vi "Populate Subpanels.vi"(8 "error in (no error)":errorcluster, 9 "View Labels (optional)":string[](array[string]), 10 "Views":refnum<class "Message Enqueuer.lvclass">[](array[class]), 11 "LeftListboxViewManager In":refnum<class "LeftListboxViewManager.lvclass">) -> (0 "error out":errorcluster, 3 "LeftListboxViewManager Out":refnum<class "LeftListboxViewManager.lvclass">)   [LabVIEW 2015, in "LeftListboxViewManager.lvlib" / "LeftListboxViewManager.lvclass"]
doc: "<License>\nCopyright © 2017 Composed Systems, LLC | All rights reserved\nwww.composed.io\n\nAuthor: Ethan Stern <ethan.stern@composed.io>\n\nThis software is provided \"AS IS\" WITHOUT WARRANTIES, either express or implied, AND IS FOR EDUCATIONAL PURPOSES ONLY.\n</License>"
uses:
  LeftListboxViewManager.lvclass
  <vilib>/ActorFramework/Message Enqueuer/Message Enqueuer.lvclass
  LeftListboxViewManager.lvclass/LeftListboxViewManager.ctl
  Framework/IViewable/IViewable Messages/Insert View Msg/Insert View Msg.lvclass/Insert View Msg.ctl
  <vilib>/ActorFramework/Message Enqueuer/Message Enqueuer.lvclass/Message Enqueuer.ctl
  <vilib>/ActorFramework/Message Enqueuer/Enqueue.vi
  <vilib>/ActorFramework/Message Priority Queue/Priority Enqueue.vi
  Framework/IViewManager/IViewManager/IViewManager.lvclass
  Framework/IViewable/IViewable Messages/Insert View Msg/Insert View Msg.lvclass
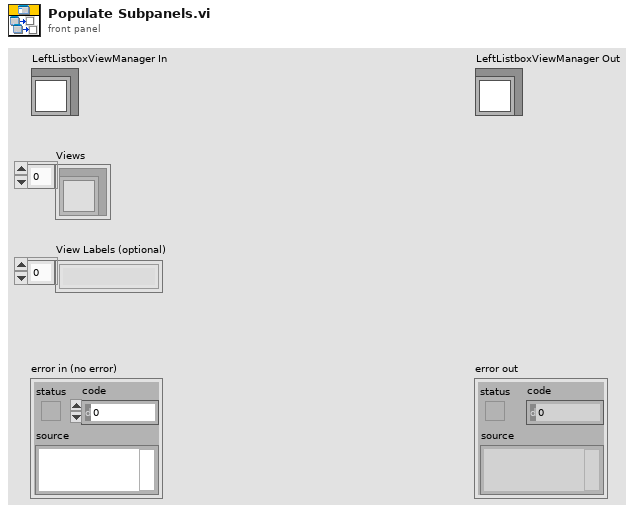
[diagram p1: front panel]
types:
  T1 = typedef "ProtectedSubpanel.lvlib/ProtectedSubpanel.lvclass/Protected Subpanel Reference.ctl" = refnum<data-value>
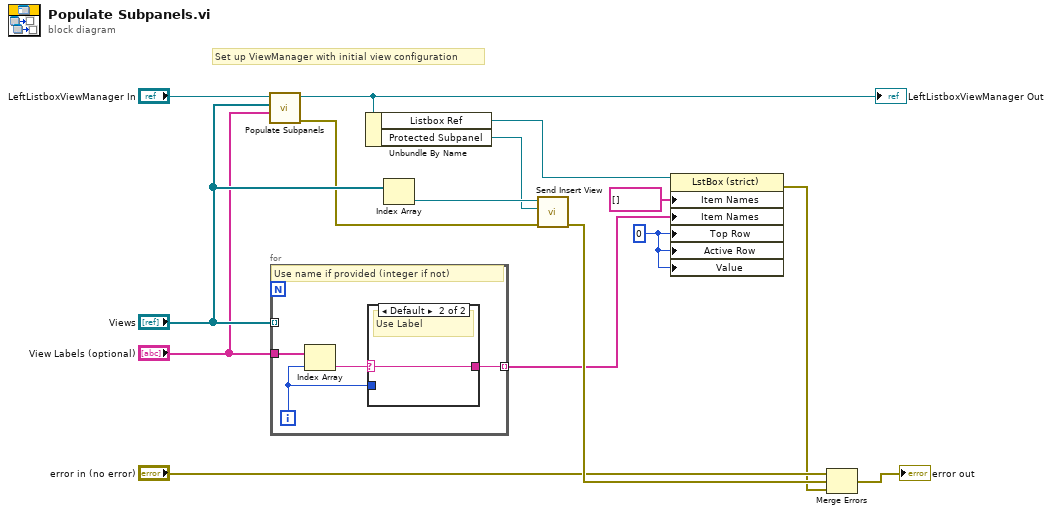
[diagram p0: block diagram]
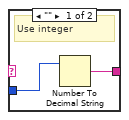
[diagram p2: hidden frame]
diagram:
  w5 = 0 ("Top Row")
  # "Set up ViewManager with initial view configuration"
  n1 = call-parent "Populate Subpanels.vi"("View Labels (optional)"="View Labels (optional)", "Views"="Views", "IViewManager In"="LeftListboxViewManager In") -> ("error out"=w2:errorcluster, "IViewManager Out"=w8:refnum<class "LeftListboxViewManager.lvclass">)  [unwired: 7 in]
  "LeftListboxViewManager Out" <- w8
  n2 = for {
    tunnel: "Views" -> [_] mode=indexing
    tunnel: "View Labels (optional)" -> [w19]
    tunnel: [w17] -> w3 mode=indexing
    i -> [w16]
    # "Use name if provided (integer if not)"
    n3 = Index Array(array=w19, index=w16) -> (element=w18:string)
    n4 = case shown="Default" w18 {
      selector: w18 -> [_ w22]
      tunnel: [w20 w22] -> w17
      tunnel: w16 -> [w21 _]
      frame "" {
        # "Use integer"
        n5 = Number To Decimal String(number=w21) -> (decimal integer string=w20:string)  [unwired: 1 in]
      }
      frame Default {
        # "Use Label"
      }
    }
  }
  n6 = Unbundle By Name(w8) -> ("Listbox Ref"=w12:refnum<vi>, "Protected Subpanel"=w13:T1)
  n7 = Index Array(array="Views") -> (element=w14:refnum<class "Message Enqueuer.lvclass">)  [unwired: 1 in]
  n8 = call "Send Insert View.vi"("error in (no error)"=w2, "Protected Subpanel"=w13, "Message Enqueuer"=w14) -> ("error out"=w10:errorcluster)  [unwired: 7 in, 1 out]
  n9 = property class="LstBox (strict)"(reference=w12, "Item Names"=string[] [], "Item Names"=w3, "Top Row"=w5, "Active Row"=w5, "Value"=w5) -> (error out=w7:errorcluster)  [unwired: 1 in, 1 out]
  n10 = Merge Errors("error in (no error)", w10, w7) -> (→"error out":errorcluster)
